vi "atm.vi"() -> ()   [LabVIEW 2018]
uses:
  <vilib>/Utility/file.llb/Read Delimited Spreadsheet (string).vi
  <vilib>/Utility/file.llb/Write Delimited Spreadsheet (string).vi
panel:
  out "选项卡控件":enum32{"选项卡 1", "选项卡 2"}(tab)
  in  "确认":bool
  in  "卡号":string
  in  "密码":string
  in  "退出":bool
  out "余额":dbl
  in  "查询":bool
  in  "存款值":dbl
  in  "存款":bool
  in  "取款值":dbl
  in  "取款":bool
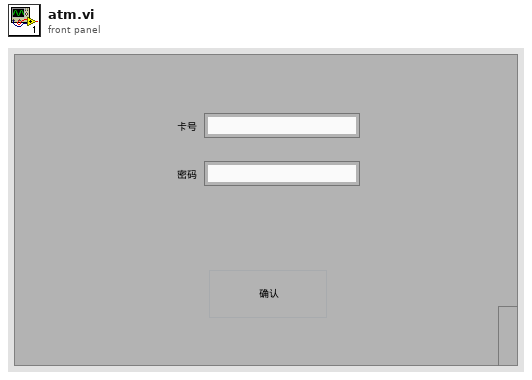
[diagram p1: front panel]
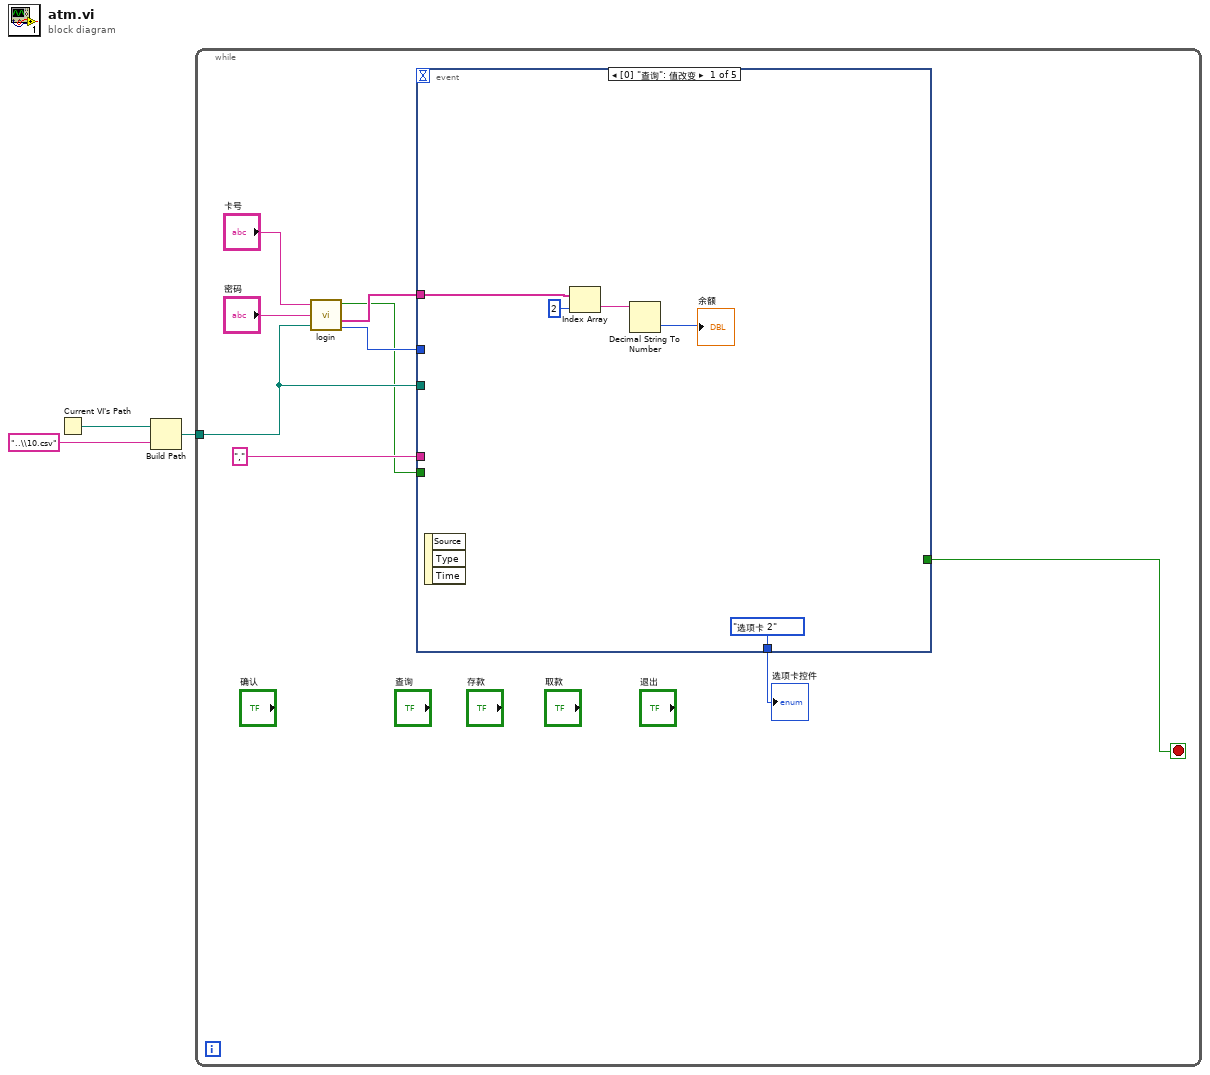
[diagram p0: block diagram]
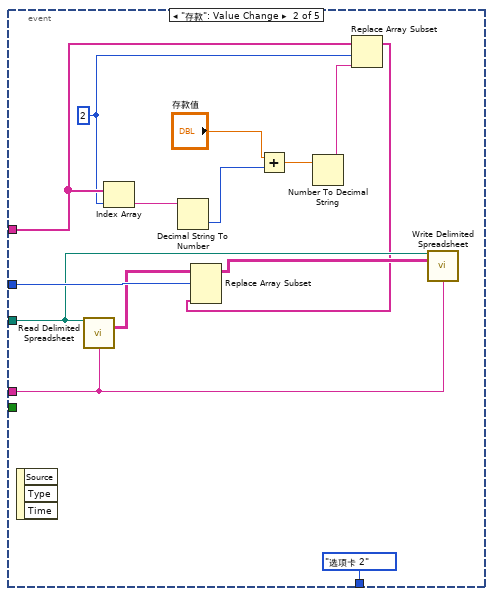
[diagram p2: hidden frame]
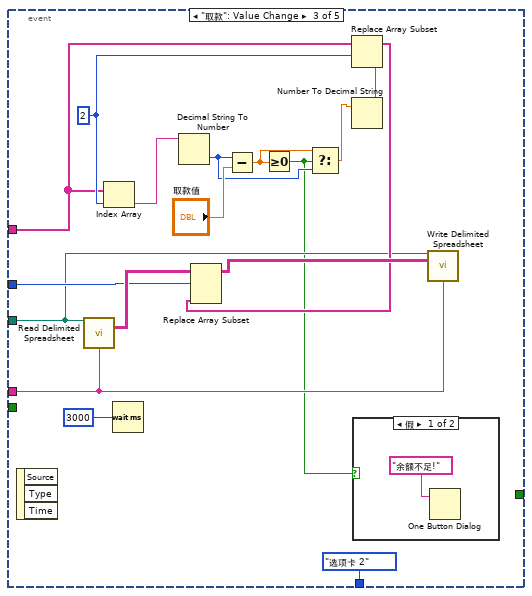
[diagram p3: hidden frame]
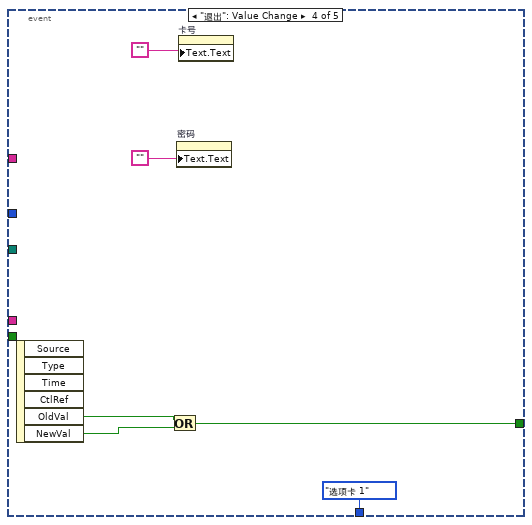
[diagram p5: hidden frame]
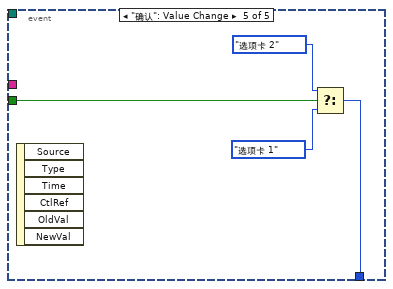
[diagram p6: hidden frame]
diagram:
  n1 = Current VI's Path() -> (path=w3:path)
  n2 = Build Path(base path=w3, name or relative path="..\\10.csv" ("delimiter (\\t)")) -> (appended path=w1:path)
  n3 = while {
    tunnel: w1 -> [w6]
    stop <- w9 stop-if-true
    n4 = call "login.vi"("卡号"="卡号", "密码"="密码", "文件"=w6) -> ("匹配"=w5:bool, "匹配信息"=w10:string[], "索引"=w7:i32)  [unwired: 1 in]
    n5 = event shown="[0] \"查询\": 值改变" {
      selector: _ -> [_ _ _ _ _]
      dyn-events: _ -> [_ _ _ _ _]
      timeout: _ -> [_ _ _ _ _]
      tunnel: w10 -> [w16 w22 w39 _ _]
      tunnel: [_ _ _ w53 _] -> w9
      tunnel: w6 -> [_ w29 w38 _ _]
      tunnel: "," ("delimiter (\\t)") -> [_ w30 w41 _ _]
      tunnel: w7 -> [_ w31 w40 _ _]
      tunnel: w5 -> [_ _ _ _ w57]
      tunnel: [enum32{"选项卡 1", "选项卡 2"}."选项卡 2" ("选项卡控件") enum32{"选项卡 1", "选项卡 2"}."选项卡 2" ("选项卡控件") enum32{"选项卡 1", "选项卡 2"}."选项卡 2" ("选项卡控件") enum32{"选项卡 1", "选项卡 2"}."选项卡 1" ("选项卡控件") w56] -> w4
      event "查询": Value Change {
        n6 = event-data() -> ()  [unwired: 1 in, 3 out]
        n7 = Index Array(array=w16, index=2 ("索引")) -> (element=w15:string)
        n8 = Decimal String To Number(string=w15) -> (number=→"余额":i32)  [unwired: 2 in, 1 out]
      }
      event "存款": Value Change {
        w21 = 2 ("索引")
        n9 = event-data() -> ()  [unwired: 1 in, 3 out]
        n10 = call-poly <vilib>:"Read Delimited Spreadsheet.vi"("file path (dialog if empty)"=w29, "delimiter (\\t)"=w30) -> ("all rows"=w26:string[][])  [unwired: 8 in, 5 out]
        n11 = Index Array(array=w22, index=w21) -> (element=w20:string)
        n12 = Decimal String To Number(string=w20) -> (number=w27:i32)  [unwired: 2 in, 1 out]
        n13 = Add(x="存款值", y=w27) -> (x+y=w24:dbl)
        n14 = Number To Decimal String(number=w24) -> (decimal integer string=w23:string)  [unwired: 1 in]
        n15 = Replace Array Subset(array=w22, new element=w23, index=w21) -> (w19:string[])
        n16 = Replace Array Subset(array=w26, new element=w19, index (row)=w31) -> (w25:string[][])  [unwired: 1 in]
        n17 = call-poly <vilib>:"Write Delimited Spreadsheet.vi"("file path (dialog if empty)"=w29, "2D data"=w25, "delimiter (\\t)"=w30) -> ()  [unwired: 11 in, 2 out]
      }
      event "取款": Value Change {
        w44 = 2 ("索引")
        n18 = event-data() -> ()  [unwired: 1 in, 3 out]
        n19 = call-poly <vilib>:"Read Delimited Spreadsheet.vi"("file path (dialog if empty)"=w38, "delimiter (\\t)"=w41) -> ("all rows"=w47:string[][])  [unwired: 8 in, 5 out]
        n20 = Index Array(array=w39, index=w44) -> (element=w43:string)
        n21 = Wait (ms)(milliseconds to wait=u32 3000 ("等待时间（毫秒）")) -> ()  [unwired: 1 out]
        n22 = Decimal String To Number(string=w43) -> (number=w34:i32)  [unwired: 2 in, 1 out]
        n23 = Subtract(x=w34, y="取款值") -> (x-y=w36:dbl)
        n24 = Greater Or Equal To 0?(x=w36) -> (x >= 0?=w33:bool)
        n25 = Select(t=w36, s=w33, f=w34) -> (s? t:f=w35:dbl)
        n26 = Number To Decimal String(number=w35) -> (decimal integer string=w45:string)  [unwired: 1 in]
        n27 = Replace Array Subset(array=w39, new element=w45, index=w44) -> (w42:string[])
        n28 = Replace Array Subset(array=w47, new element=w42, index (row)=w40) -> (w46:string[][])  [unwired: 1 in]
        n29 = case shown="假" w33 {
          frame False {
            n30 = One Button Dialog(message="余额不足!" ("消息")) -> ()  [unwired: 1 in, 1 out]
          }
          frame True {
          }
        }
        n31 = call-poly <vilib>:"Write Delimited Spreadsheet.vi"("file path (dialog if empty)"=w38, "2D data"=w46, "delimiter (\\t)"=w41) -> ()  [unwired: 11 in, 2 out]
      }
      event "退出": Value Change {
        n32 = event-data() -> ("OldVal"=w55:bool, "NewVal"=w54:bool)  [unwired: 1 in, 4 out]
        n33 = Or(x=w55, y=w54) -> (x .or. y?=w53:bool)
        n34 = property on="密码" class="Str"("Text.Text"="") -> ()  [unwired: 2 in, 2 out]
        n35 = property on="卡号" class="Str"("Text.Text"="") -> ()  [unwired: 2 in, 2 out]
      }
      event "确认": Value Change {
        n36 = event-data() -> ()  [unwired: 1 in, 6 out]
        n37 = Select(t=enum32{"选项卡 1", "选项卡 2"}."选项卡 2" ("选项卡控件"), s=w57, f=enum32{"选项卡 1", "选项卡 2"}."选项卡 1" ("选项卡控件")) -> (s? t:f=w56:enum32{"选项卡 1", "选项卡 2"})
      }
    }
    "选项卡控件" <- w4
  }
